vi "Stat Bundles to Table.vi"(0 "StatBundle":T1(array[cluster])) -> (4 "table.Stats":string[][](array[string]))   [LabVIEW 2019]
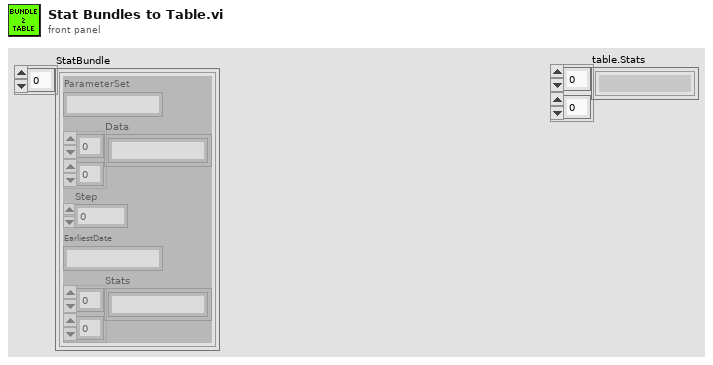
[diagram p1: front panel]
types:
  T1 = cluster{"ParameterSet":string, "Data":string[][], "Step":i32, "EarliestDate":string, "Stats":string[][]}[]
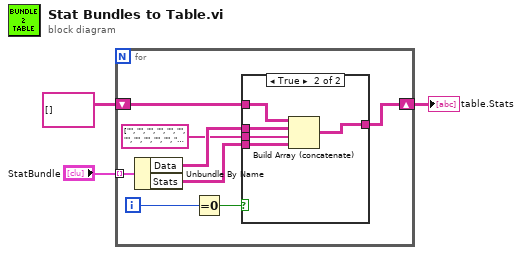
[diagram p0: block diagram]
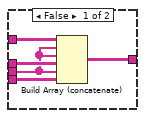
[diagram p2: hidden frame]
diagram:
  n1 = for {
    shift-right: [w4] -> w1
    shift-left: string[][] [] -> [w10]
    tunnel: "StatBundle" -> [w11] mode=indexing
    i -> [w9]
    n2 = Unbundle By Name(w11) -> ("Data"=w7:string[][], "Stats"=w6:string[][])
    n3 = Equal To 0?(x=w9) -> (x = 0?=w8:bool)
    n4 = case shown="True" w8 {
      tunnel: w10 -> [w16 w21]
      tunnel: w7 -> [w15 w18]
      tunnel: w6 -> [w14 w20]
      tunnel: string[] ["", "", "", "", "", "", "", "", "", "", "", "", "", ""] -> [w13 w19]
      tunnel: [w12 w17] -> w4
      frame False {
        n5 = Build Array (concatenate)(w16, w13, w13, w15, w13, w14) -> (w12:string[][])
      }
      frame True {
        n6 = Build Array (concatenate)(w21, w18, w19, w20) -> (w17:string[][])
      }
    }
  }
  "table.Stats" <- w1
